vi "test Timestamp Added To File Name.vi"(8 "error in (no error)":errorcluster, 11 "TestCase in":refnum<class "Build Linux Log File Path.lvclass">) -> (0 "error out":errorcluster, 3 "TestCase out":refnum<class "Build Linux Log File Path.lvclass">)   [LabVIEW 2024, in "Build Linux Log File Path.lvclass"]
uses:
  Build Linux Log File Path.lvclass
  <vilib>/regexp/Match Regular Expression.xnode
  <vilib>/addons/_JKI Toolkits/VI Tester/TestCase.llb/TestCase.lvclass
  C:/Program Files/National Instruments/LabVIEW 2024/vi.lib/addons/_JKI Toolkits/VI Tester/TestCase.llb/TestCase.lvclass
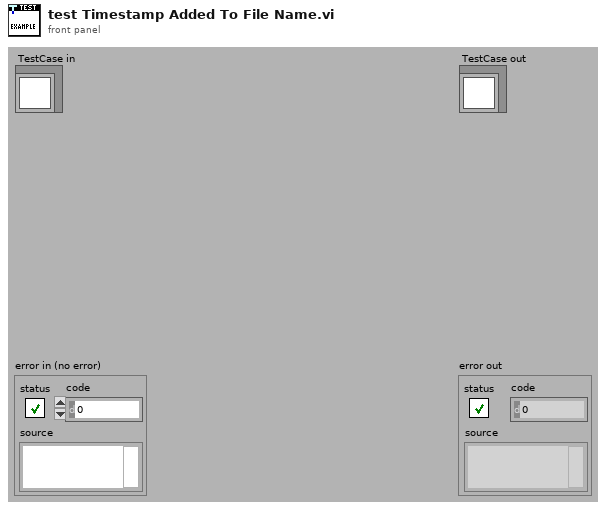
[diagram p1: front panel]
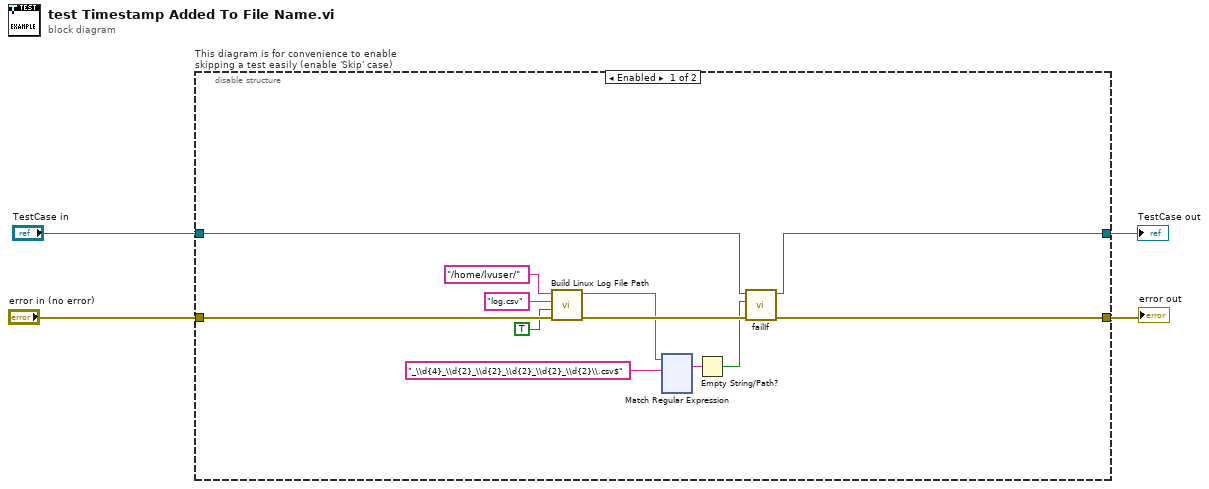
[diagram p0: block diagram]
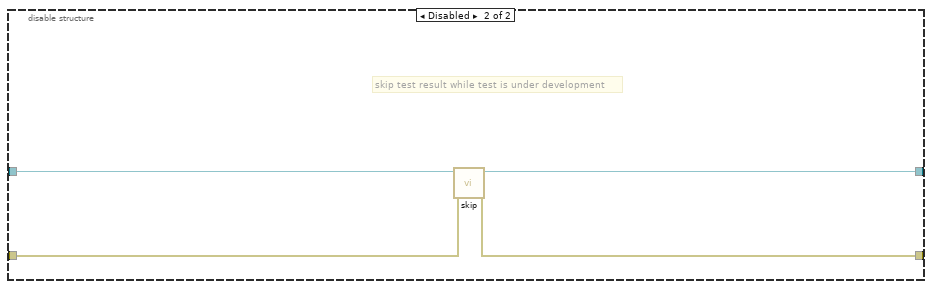
[diagram p2: hidden frame]
diagram:
  n1 = disable-structure "This diagram is for convenience to enable skipping a test easily (enable 'Skip' case)" shown="Enabled" {
    disable-tunnel: "TestCase in" -> [w15 w137]
    disable-tunnel: [w10 w135] -> w1
    disable-tunnel: [w9 w136] -> w3
    disable-tunnel: "error in (no error)" -> [w16 w134]
    frame Enabled {
      n2 = call "Build Linux Log File Path.vi"("error in (no error)"=w16, "Timestamp"=TRUE, "Name"="log.csv", "Log File Directory"="/home/lvuser/") -> ("error out"=w14:errorcluster, "Log File Path"=w8:string)  [unwired: 6 in]
      n3 = xnode "Match Regular Expression"("input string"=w8, "regular expression"="_\\d{4}_\\d{2}_\\d{2}_\\d{2}_\\d{2}_\\d{2}\\.csv$") -> ("whole match"=w6:string)  [unwired: 4 in, 4 out]
      n4 = Empty String/Path?(string/path=w6) -> (empty?=w5:bool)
      n5 = call-dynamic "failIf.vi"("error in (no error)"=w14, "fail"=w5, "TestCase in"=w15) -> ("error out"=w9:errorcluster, "TestCase out"=w10:refnum<class "Build Linux Log File Path.lvclass">)  [unwired: 7 in]
    }
    frame Disabled {
      # "skip test result while test is under development"
      n6 = call <vilib>:"skip.vi"("error in (no error)"=w134, "TestCase in"=w137) -> ("error out"=w136:errorcluster, "TestCase out"=w135:refnum<class "Build Linux Log File Path.lvclass">)  [unwired: 8 in]
    }
  }
  "error out" <- w3
  "TestCase out" <- w1
